vi "Create Counter Driven Output Channel.vi"(6 "index":i32, 7 "counter driven state":T1, 8 "error in":errorcluster, 9 "default value":bool, 10 "name":string, 11 "counter driven output channel in":refnum<class "Counter Driven Output Channel.lvclass">) -> (0 "error out":errorcluster, 3 "counter driven output channel out":refnum<class "Counter Driven Output Channel.lvclass">)   [LabVIEW 2020, in "Scan Engine Scripting.lvlib" / "Counter Driven Output Channel.lvclass"]
uses:
  Counter Driven Output Channel.lvclass
  Counter Driven State.ctl
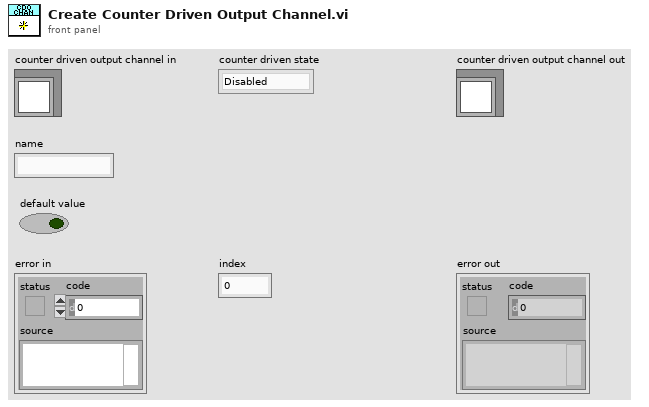
[diagram p1: front panel]
types:
  T1 = typedef "Scan Engine Scripting.lvlib/Counter Driven Output Channel.lvclass/Counter Driven State.ctl" = enum16{"Disabled", "Enabled"}
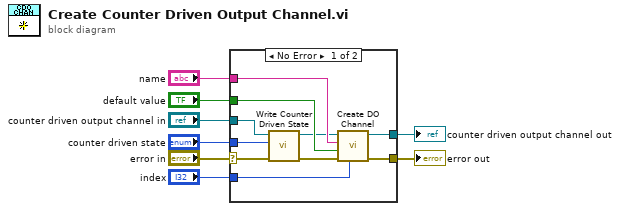
[diagram p0: block diagram]
diagram:
  n1 = case shown="No Error" "error in" {
    selector: "error in" -> [w9 w19]
    tunnel: "counter driven state" -> [w18 _]
    tunnel: "name" -> [w17 _]
    tunnel: "default value" -> [w16 _]
    tunnel: "index" -> [w15 _]
    tunnel: [w13 w20] -> w4
    tunnel: [w11 w19] -> w3
    tunnel: "counter driven output channel in" -> [w10 w20]
    frame No Error {
      n2 = call-dynamic "Write Counter Driven State.vi"("error in"=w9, "counter driven state"=w18, "counter driven output channel in"=w10) -> ("error out"=w12:errorcluster, "counter driven output channel out"=w14:refnum<class "Counter Driven Output Channel.lvclass">)  [unwired: 7 in]
      n3 = call-dynamic "Create DO Channel.vi"("index"=w15, "error in"=w12, "default value"=w16, "name"=w17, "DO channel in"=w14) -> ("error out"=w11:errorcluster, "DO channel out"=w13:refnum<class "Counter Driven Output Channel.lvclass">)  [unwired: 5 in]
    }
    frame Error {
    }
  }
  "error out" <- w3
  "counter driven output channel out" <- w4
